vi "AD5781.vi"(8 "Send":bool=TRUE) -> (0 "Readback":u32 format="%024b", 1 "Readback 0":u32 format="%032b", 3 "DACtimeOut":bool)   [LabVIEW 2014]
uses:
  <vilib>/rvi/Emulation/niFpgaGetClockAttributes.vi
  <vilib>/rvi/Emulation/niFpgaSctlEmulationGetInTimedLoop.vi
  <vilib>/rvi/Emulation/niFpgaEmulationReportErrorSimple.vi
  Code/FPGA SPI_Globals.vi
  <vilib>/rvi/Emulation/niFpgaProcessEmulError.vi
  <vilib>/rvi/Emulation/niFpgaCriticalErrorInLSC.vi
  SimpleCounter/SCGlobVars.vi
panel:
  in  "SetVolt":u32 format="%024b"
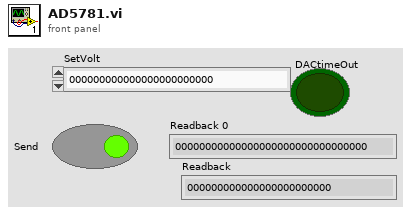
[diagram p1: front panel]
types:
  T1 = cluster{"SCLK":refnum<k21>, "CS":refnum<k21>, "MOSI":refnum<k21>, "MISO":refnum<k21>}
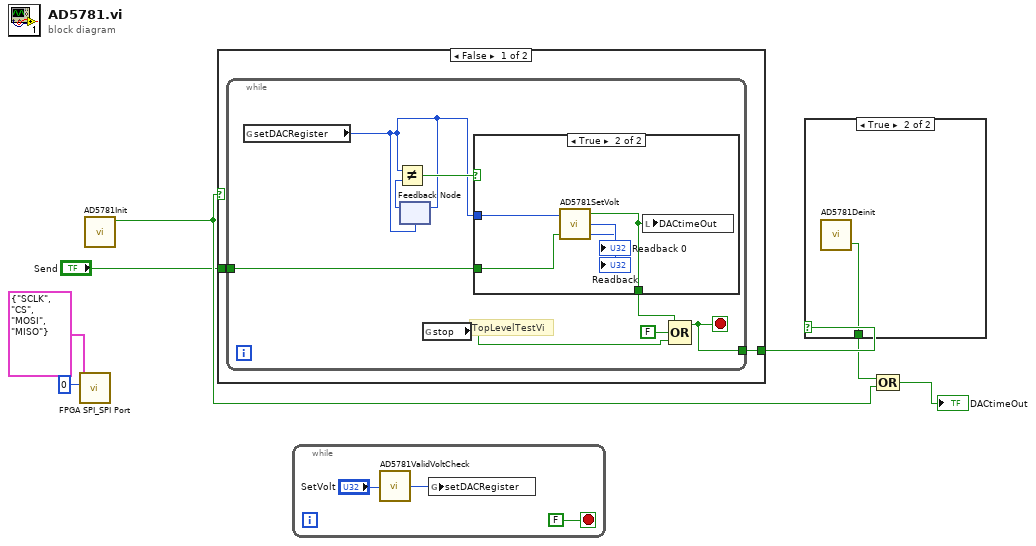
[diagram p0: block diagram]
diagram:
  # "TopLevelTestVi"
  n1 = call "FPGA SPI_SPI Port.vi"("Port"=i8 0, "FPGA IO"=T1 {"SCLK"="SCLK", "CS"="CS", "MOSI"="MOSI", "MISO"="MISO"}) -> ()  [unwired: 10 in]
  n2 = call "AD5781Init.vi"() -> ("timeOut"=w4:bool)  [unwired: 11 in]
  n3 = case shown="False" w4 {
    tunnel: [w9 _] -> w5
    tunnel: "Send" -> [w8 _]
    frame False {
      n4 = while {
        tunnel: [w13] -> w9
        tunnel: w8 -> [w11]
        stop <- w13 stop-if-true
        n5 = global read "FPGA SPI_Globals.vi" "setDACRegister"() -> (w10:u32)
        n6 = feedback-in #1(w10) -> ()
        n7 = feedback #1(w10) -> (w15:u32)
        n8 = Not Equal?(x=w10, y=w15) -> (x != y?=w14:bool)
        n9 = global read "SCGlobVars.vi" "stop"() -> (w12:bool)
        n10 = case shown="True" w14 {
          tunnel: w10 -> [_ w22]
          tunnel: [_ w21] -> w16
          tunnel: w11 -> [_ w18]
          frame False {
          }
          frame True {
            n11 = call "AD5781SetVolt.vi"("Send"=w18, "SetVolt"=w22) -> ("Readback"=→"Readback":u32, "Readback 0"=→"Readback 0":u32, "timedOut"=w21:bool)  [unwired: 1 in]
            n12 = local write "DACtimeOut"(w21) -> ()
          }
        }
        n13 = Compound Arithmetic op=OR(w16, FALSE, w12) -> (w13:bool)
      }
    }
    frame True {
    }
  }
  n14 = while {
    stop <- FALSE stop-if-true
    n15 = call "AD5781ValidVoltCheck.vi"("U32"="SetVolt") -> ("coerced(x)"=w23:u32)  [unwired: 4 in]
    n16 = global write "FPGA SPI_Globals.vi" "setDACRegister"(w23) -> ()
  }
  n17 = case shown="True" w5 {
    tunnel: [_ w26] -> w2
    frame False {
    }
    frame True {
      n18 = call "AD5781Deinit.vi"() -> ("timedOut"=w26:bool)  [unwired: 3 in]
    }
  }
  n19 = Compound Arithmetic op=OR(w2, w4) -> (→"DACtimeOut":bool)
